vi "json_makeControl.vi"(8 "error in (no error)":errorcluster) -> (0 "error out":errorcluster, 3 "ctl ref":refnum<vi>)   [LabVIEW 2011]
doc: "Creates a ctl."
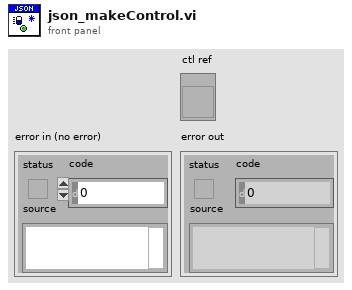
[diagram p1: front panel]
types:
  T1 = enum32{"not a control VI", "control", "typedef", "strict typedef"}
  T2 = enum32{"invalid VI type", "Standard VI", "Control VI", "Global VI", "Polymorphic VI", "Configuration VI", "SubSystem", "Facade VI", "Method VI", "Statechart Diagram VI"}
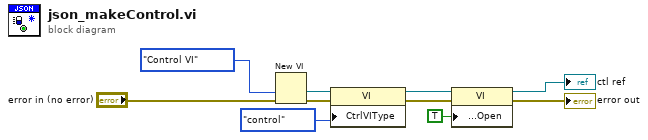
[diagram p0: block diagram]
diagram:
  n1 = New VI(8:"error in (no error)", 9:T2."Control VI" ("vi type (standard vi)")) -> (0:w9:errorcluster, 3:w8:refnum<vi>)  [unwired: 5 in]
  n2 = property class="VI"(reference=w8, error in=w9, "CtrlVIType"=T1."control" ("Control VI Type")) -> (reference out=w6:refnum<vi>, error out=w5:errorcluster)
  n3 = property class="VI"(reference=w6, error in=w5, "Front Panel.Open"=TRUE ("Front Panel Window:Open")) -> (reference out=→"ctl ref":refnum<vi>, error out=→"error out":errorcluster)
